vi "loginScreenCoklu.vi"() -> ()   [LabVIEW 2015]
uses:
  <vilib>/regexp/Match Regular Expression.xnode
panel:
  out "led":bool
  in  "OK Button":bool
  in  "password":string
  in  "user name":string
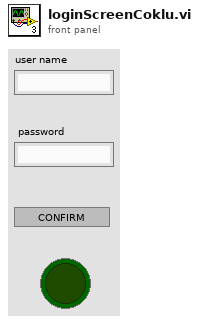
[diagram p1: front panel]
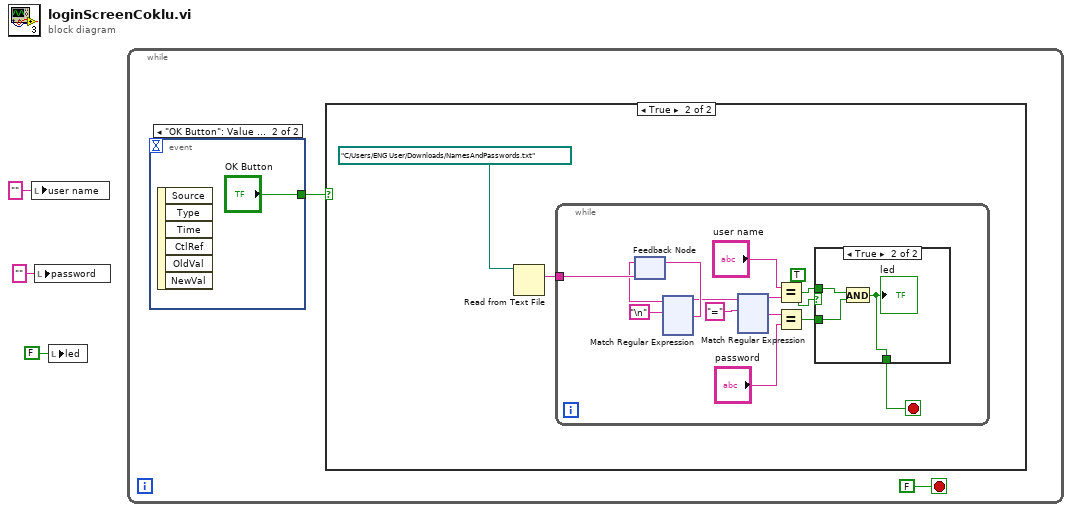
[diagram p0: block diagram]
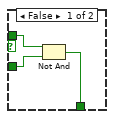
[diagram p3: hidden frame]
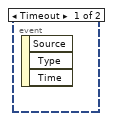
[diagram p4: hidden frame]
diagram:
  n1 = local write "user name"("" ("user name")) -> ()
  n2 = local write "password"("" ("password")) -> ()
  n3 = local write "led"(FALSE ("led")) -> ()
  n4 = while {
    stop <- FALSE stop-if-true
    n5 = event shown="[1] \"OK Button\": Value Change" {
      selector: _ -> [_ _]
      dyn-events: _ -> [_ _]
      timeout: _ -> [_ _]
      tunnel: [_ "OK Button"] -> w5
      event Timeout {
        n6 = event-data() -> ()  [unwired: 1 in, 3 out]
      }
      event "OK Button": Value Change {
        n7 = event-data() -> ()  [unwired: 1 in, 6 out]
      }
    }
    n8 = case shown="True" w5 {
      frame False {
      }
      frame True {
        n9 = Read from Text File(file (use dialog)=path "C:/Users/ENG User/Downloads/NamesAndPasswords.txt" ("text")) -> (text=w7:string)  [unwired: 3 in, 3 out]
        n10 = while {
          tunnel: w7 -> [w21]
          stop <- w9 stop-if-true
          n11 = feedback #1(w21) -> (w20:string)
          n12 = xnode ("Match Regular Expression")("input string"=w20, "regular expression"="\n" ("Line Feed Constant")) -> ("before match"=w17:string, "after match"=w19:string)  [unwired: 4 in, 3 out]
          n13 = feedback-in #1(w19) -> ()
          n14 = xnode ("Match Regular Expression")("input string"=w17, "regular expression"="=") -> ("before match"=w15:string, "after match"=w13:string)  [unwired: 4 in, 3 out]
          n15 = Equal?(x="user name", y=w15) -> (x = y?=w11:bool)
          n16 = Equal?(x=w13, y="password") -> (x = y?=w10:bool)
          n17 = case shown="True" TRUE {
            tunnel: w11 -> [w24 w27]
            tunnel: w10 -> [w23 w26]
            tunnel: [w22 w25] -> w9
            frame False {
              n18 = Not And(1:w23, 2:w24) -> (0:w22:bool)
            }
            frame True {
              n19 = And(x=w27, y=w26) -> (x .and. y?=w25:bool)
              "led" <- w25
            }
          }
        }
      }
    }
  }
